vi "PID Get Advanced Error (DBL Array).vi"(0 "error buffer":dbl[](array[numeric]) format="%.2f", 1 "setpoint":dbl[](array[numeric])=[0.0] format="%.2f", 2 "beta":dbl[](array[numeric])=[1.0] format="%.2f", 3 "linearity":dbl[](array[numeric])=[1.0] format="%.2f", 5 "error (with beta) buffer":dbl[](array[numeric]) format="%.2f", 7 "non-linear integral buffer":dbl[](array[numeric]) format="%.2f", 9 "process variable":dbl[](array[numeric])=[0.0] format="%.2f", 10 "process variable size":i32, 11 "error (with gamma) buffer":dbl[](array[numeric]) format="%.2f", 12 "setpoint range":T1(array[cluster])=[{"setpoint high"=100.0, "setpoint low"=0.0}] {"setpoint high" format="%.2f"; "setpoint low" format="%.2f"}, 13 "gamma":dbl[](array[numeric])=[0.0] format="%.2f", 14 "Kp":dbl[](array[numeric])) -> (4 "error":dbl[](array[numeric]) format="%.2f", 6 "error (with beta)":dbl[](array[numeric]) format="%.2f", 8 "non-linear integral":dbl[](array[numeric]) format="%.2f", 15 "error (with gamma)":dbl[](array[numeric]) format="%.2f")   [LabVIEW 2017, in "NI_PID_pid.lvlib"]
doc: "This function calculates the error between the process variable and setpoint value. The error (with beta) output is used for the proportional action and the error output is used for the integral action."
uses:
  <vilib>/addons/control/pid/NI_PID_pid.lvlib
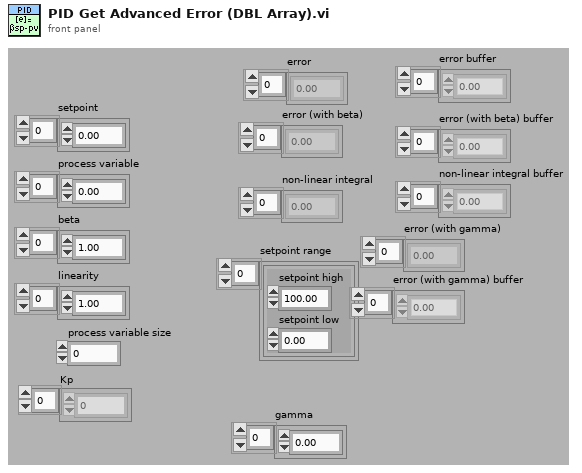
[diagram p1: front panel]
types:
  T1 = cluster{"setpoint high":dbl, "setpoint low":dbl}[]
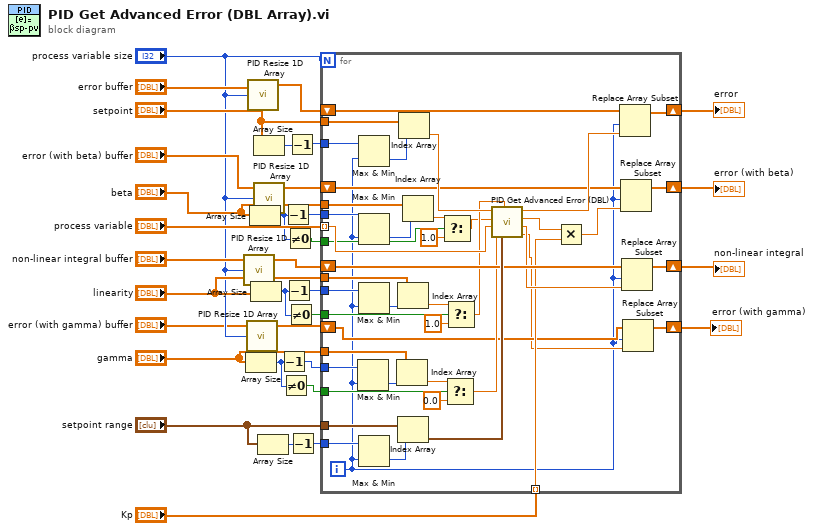
[diagram p0: block diagram]
diagram:
  n1 = call <vilib>:"PID Resize 1D Array.vi"("array size"="process variable size", "input array"="non-linear integral buffer") -> ("output array"=w20:dbl[])  [unwired: 3 out]
  n2 = Array Size(array="gamma") -> (size(s)=w5:i32)
  n3 = call <vilib>:"PID Resize 1D Array.vi"("array size"="process variable size", "input array"="error (with gamma) buffer") -> ("output array"=w2:dbl[])  [unwired: 3 out]
  n4 = call <vilib>:"PID Resize 1D Array.vi"("array size"="process variable size", "input array"="error buffer") -> ("output array"=w9:dbl[])  [unwired: 3 out]
  n5 = Array Size(array="beta") -> (size(s)=w17:i32)
  n6 = Array Size(array="linearity") -> (size(s)=w23:i32)
  n7 = Array Size(array="setpoint") -> (size(s)=w13:i32)
  n8 = call <vilib>:"PID Resize 1D Array.vi"("array size"="process variable size", "input array"="error (with beta) buffer") -> ("output array"=w18:dbl[])  [unwired: 3 out]
  n9 = Array Size(array="setpoint range") -> (size(s)=w30:i32)
  n10 = Decrement(x=w5) -> (x-1=w8:i32)
  n11 = Not Equal To 0?(x=w5) -> (x != 0?=w7:bool)
  n12 = Decrement(x=w17) -> (x-1=w16:i32)
  n13 = Decrement(x=w23) -> (x-1=w27:i32)
  n14 = Not Equal To 0?(x=w17) -> (x != 0?=w14:bool)
  n15 = Not Equal To 0?(x=w23) -> (x != 0?=w22:bool)
  n16 = Decrement(x=w13) -> (x-1=w12:i32)
  n17 = Decrement(x=w30) -> (x-1=w28:i32)
  n18 = for {
    N: "process variable size" -> [_]
    tunnel: "process variable" -> [w73] mode=indexing
    tunnel: "setpoint range" -> [w77]
    tunnel: w28 -> [w76]
    tunnel: w27 -> [w74]
    shift-right: [w69] -> w31
    shift-left: w9 -> [w70]
    shift-right: [w67] -> w32
    shift-left: w18 -> [w66]
    shift-right: [w64] -> w26
    shift-left: w20 -> [w65]
    tunnel: "Kp" -> [w60] mode=indexing
    tunnel: "linearity" -> [w59]
    tunnel: w22 -> [w56]
    tunnel: w16 -> [w54]
    tunnel: "beta" -> [w52]
    tunnel: w14 -> [w49]
    tunnel: w12 -> [w47]
    tunnel: "setpoint" -> [w45]
    tunnel: w8 -> [w41]
    tunnel: w7 -> [w40]
    tunnel: "gamma" -> [w39]
    shift-right: [w37] -> w3
    shift-left: w2 -> [w36]
    i -> [w34]
    n19 = Max & Min(x=w41, y=w34) -> (min(x,y)=w42:i32)  [unwired: 1 out]
    n20 = Max & Min(x=w47, y=w34) -> (min(x,y)=w46:i32)  [unwired: 1 out]
    n21 = Max & Min(x=w54, y=w34) -> (min(x,y)=w53:i32)  [unwired: 1 out]
    n22 = Max & Min(x=w74, y=w34) -> (min(x,y)=w75:i32)  [unwired: 1 out]
    n23 = Max & Min(x=w76, y=w34) -> (min(x,y)=w78:i32)  [unwired: 1 out]
    n24 = Index Array(array=w39, index=w42) -> (element=w43:dbl)
    n25 = Index Array(array=w59, index=w75) -> (element=w58:dbl)
    n26 = Index Array(array=w77, index=w78) -> (element=w72:cluster{"setpoint high":dbl, "setpoint low":dbl})
    n27 = Index Array(array=w45, index=w46) -> (element=w71:dbl)
    n28 = Index Array(array=w52, index=w53) -> (element=w50:dbl)
    n29 = Select(t=w50, s=w49, f=1.0) -> (s? t:f=w48:dbl)
    n30 = Select(t=w43, s=w40, f=0.0) -> (s? t:f=w38:dbl)
    n31 = Select(t=w58, s=w56, f=1.0) -> (s? t:f=w57:dbl)
    n32 = call <vilib>:"PID Get Advanced Error (DBL).vi"("setpoint range"=w72, "linearity"=w57, "Gamma"=w38, "process variable"=w73, "beta"=w48, "setpoint"=w71) -> ("error with gamma"=w35:dbl, "non-linear integral action"=w63:dbl, "error with beta"=w61:dbl, "error"=w68:dbl)  [unwired: 2 out]
    n33 = Multiply(x=w61, y=w60) -> (x*y=w62:dbl)
    n34 = Replace Array Subset(array=w70, new element=w68, index=w34) -> (w69:dbl[])
    n35 = Replace Array Subset(array=w66, new element=w62, index=w34) -> (w67:dbl[])
    n36 = Replace Array Subset(array=w65, new element=w63, index=w34) -> (w64:dbl[])
    n37 = Replace Array Subset(array=w36, new element=w35, index=w34) -> (w37:dbl[])
  }
  "error" <- w31
  "error (with beta)" <- w32
  "non-linear integral" <- w26
  "error (with gamma)" <- w3
